vi "ingest.mcap_add_file_tag.vi"(8 "error in":errorcluster, 11 "McapIngestStaging in":refnum<class "McapIngestStaging.lvclass">) -> (0 "error out":errorcluster, 3 "McapIngestStaging out":refnum<class "McapIngestStaging.lvclass">)   [LabVIEW 2020, in "McapIngestStaging.lvclass"]
doc: "Applies a fixed tag and value to every record ingested from the MCAP file."
uses:
  McapIngestStaging.lvclass
  McapIngestStaging.lvclass/McapIngestStaging.ctl
  client.lvlib
panel:
  in  "tag":string
  in  "value":string
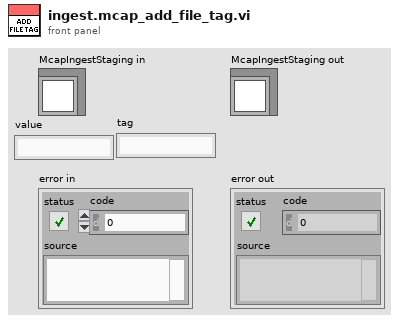
[diagram p1: front panel]
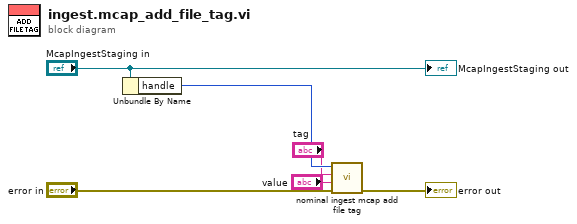
[diagram p0: block diagram]
diagram:
  n1 = Unbundle By Name("McapIngestStaging in") -> ("handle"=w4:i32)
  n2 = call "nominal ingest mcap add file tag.vi"("error in (no error)"="error in", "value"="value", "tag"="tag", "staging"=w4) -> ("error out"=→"error out":errorcluster)  [unwired: 6 in, 1 out]
  "McapIngestStaging out" <- "McapIngestStaging in"
